vi "EOMSettings.vi"(1 "Get/Set":bool, 2 "EOM Settings (input)":T1={"Output Channel"="1", "EOM Voltage"=10.0, "Pixel per Polymode Cycle"=10, "Time per Polymode Cycle"=5.0} {"Time per Polymode Cycle" format="%.2f"; "Pixel per Polymode Cycle" max=20 step=1; "EOM Voltage" min=0.0 max=20.0 step=1.0 format="%.2f"}) -> (0 "EOM Settings (output)":T1={"Output Channel"="1", "EOM Voltage"=10.0, "Pixel per Polymode Cycle"=10, "Time per Polymode Cycle"=5.0} {"Time per Polymode Cycle" format="%.2f"; "Pixel per Polymode Cycle" max=20 step=1; "EOM Voltage" min=0.0 max=20.0 step=1.0 format="%.2f"})   [LabVIEW 2009]
uses:
  EOMSettings.ctt
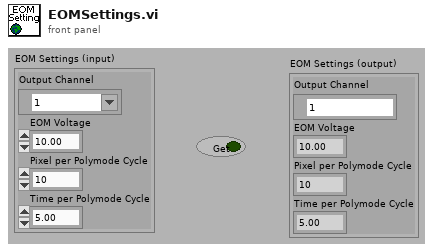
[diagram p1: front panel]
types:
  T1 = typedef "EOMSettings.ctt" = cluster{"Output Channel":tag, "EOM Voltage":dbl, "Pixel per Polymode Cycle":u32, "Time per Polymode Cycle":dbl}
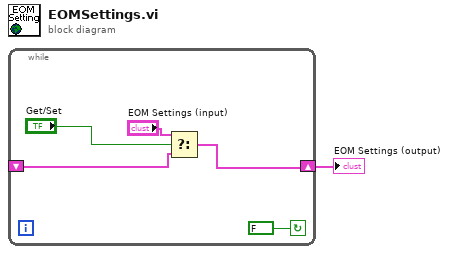
[diagram p0: block diagram]
diagram:
  n1 = while {
    shift-right: [w3] -> w1
    shift-left: _ -> [w4]
    stop <- FALSE continue-if-true
    n2 = Select(t="EOM Settings (input)", s="Get/Set", f=w4) -> (s? t:f=w3:T1)
  }
  "EOM Settings (output)" <- w1
